vi "DisplaySubscriber.vi"(11 "CSV Input":string) -> (1 "CSV output":string, 3 "Published Data":string[][](array[string]))   [LabVIEW 2015]
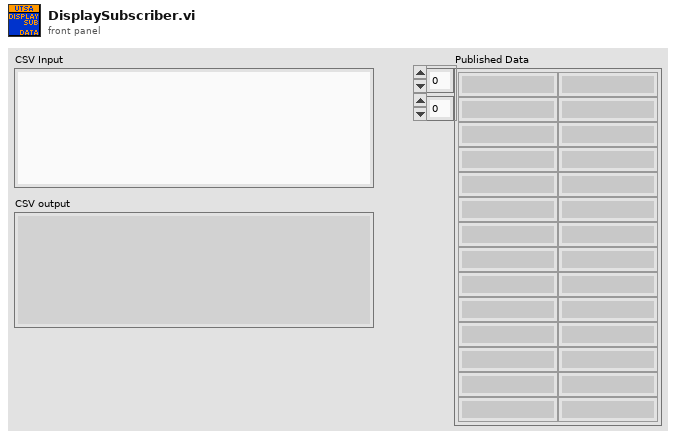
[diagram p1: front panel]
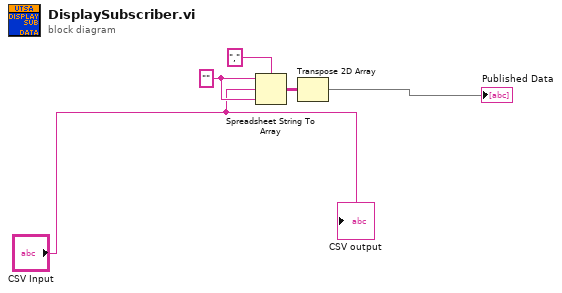
[diagram p0: block diagram]
diagram:
  w4 = "" ("format string")
  n1 = Spreadsheet String To Array(delimiter (Tab)=",", format string=w4, spreadsheet string="CSV Input", array type (2D Dbl)=w4) -> (array=w3:string[][])
  n2 = Transpose 2D Array(2D array=w3) -> (transposed array=→"Published Data":string[][])
  "CSV output" <- "CSV Input"
